vi "initialize Session Data.vi"(0 "OBJ - Session in":refnum<class "Config Data.lvclass">, 11 "error in":errorcluster) -> (4 "OBJ - Session out":refnum<class "Config Data.lvclass">, 15 "error out":errorcluster)   [LabVIEW 2014, in "Config Data.lvclass"]
doc: "OVERRIDE VI\nPlaceholder for decendant sessions to initialize and set their default values"
uses:
  Config Data.lvclass
  Config Data.lvclass/Config Data.ctl
  Accessors/Read Cfg Path.vi
  Accessors/Write Ref.vi
  <vilib>/Utility/config.llb/NI_LVConfig.lvlib
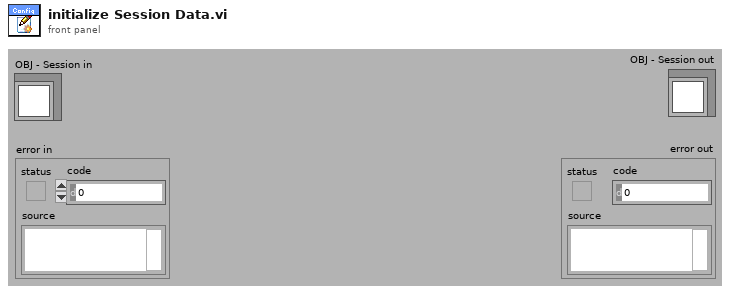
[diagram p1: front panel]
types:
  T1 = typedef "NI_LVConfig.lvlib/Config Data RefNum.ctl" = refnum<k1>
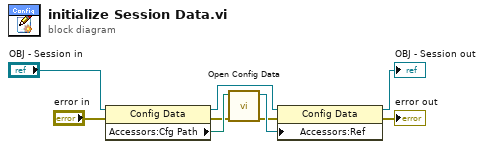
[diagram p0: block diagram]
diagram:
  n1 = property class="Config Data"(reference="OBJ - Session in", error in="error in") -> (reference out=w7:refnum<class "Config Data.lvclass">, error out=w2:errorcluster, "Accessors:Cfg Path"=w8:path)
  n2 = call <vilib>:"Open Config Data.vi"("error in (no error)"=w2, "configuration file path"=w8) -> ("error out"=w1:errorcluster, "refnum"=w6:T1)  [unwired: 7 in, 1 out]
  n3 = property class="Config Data"(reference=w7, error in=w1, "Accessors:Ref"=w6) -> (reference out=→"OBJ - Session out":refnum<class "Config Data.lvclass">, error out=→"error out":errorcluster)
